vi "Destroy.vi"(0 "reference in":refnum<class "Logger.lvclass">, 5 "Error In":errorcluster) -> (14 "reference out":refnum<class "Logger.lvclass">, 19 "Error Out":errorcluster)   [LabVIEW 2023, in "Logger.lvclass"]
uses:
  Logger.lvclass
  Logger.lvclass/Logger.ctl
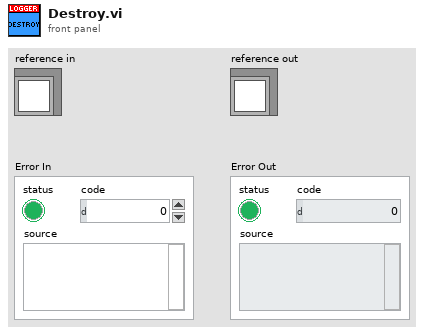
[diagram p1: front panel]
types:
  T1 = typedef "VI-TechBaseTemplate_Simple_6x8x6.lvclass/ObjectAttributes.ctl" = cluster{"Attribute1":dbl}
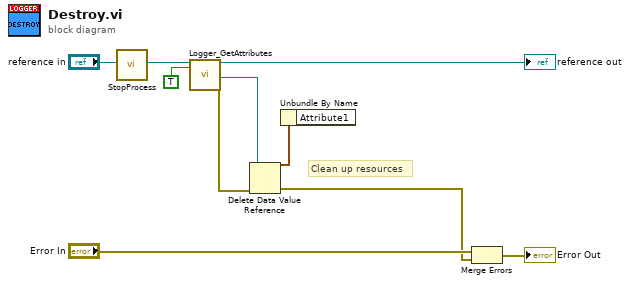
[diagram p0: block diagram]
diagram:
  # "Clean up resources"
  n1 = call "StopProcess.vi"("reference in"="reference in") -> ("reference out"=w1:refnum<class "Logger.lvclass">)  [unwired: 17 in, 1 out]
  n2 = call "Logger_GetAttributes.vi"("reference in"=w1, "OnlyGetDvrReference(False)"=TRUE) -> ("reference out"=→"reference out":refnum<class "Logger.lvclass">, "DataRef"=w7:refnum<data-value>, "Error Out"=w8:errorcluster)  [unwired: 14 in, 1 out]
  n3 = Delete Data Value Reference(data value reference=w7, error in=w8) -> (data value=w3:T1, error out=w5:errorcluster)
  n4 = Unbundle By Name(w3) -> ()  [unwired: 1 out]
  n5 = Merge Errors("Error In", w5) -> (→"Error Out":errorcluster)
